vi "1-Continuous B sweep.vi"(2 "Comments":string="SA03036H\nsweep Vsg:-150m to 700m, 500u steps\nB 7T to -7T\nVbg =-3.9V\nT: 50mK\n\nlockin\n\nI+/-: 4/28 200uV ac+ 250u dc bias, 13Hz\nV1+/-: 3/27\nV2+/- 2/6\nV3+/V3-: 7/8\nVsg: 1\nVbg :26\n\ntc 300ms order 2", 3 "ITX folder":string="4L4Lockinfieldsweep", 5 "Sweep rate (T/min)":dbl=0.028 min=0.0 max=0.2, 6 "error in (no error)":errorcluster, 7 "Simulate/Run":enum16{"simulate mode", "run mode"}(ring)=enum."run mode", 8 "Min (start)":dbl=7.0 min=-8.0 max=8.0, 9 "Max (end)":dbl=-7.0 min=-8.0 max=8.0) -> (0 "error out":errorcluster)   [LabVIEW 2016, in "Transport.lvclass"]
uses:
  Transport.lvclass
  SMOs/SweepControl/SweepControl.lvclass
  C:/Program Files (x86)/National Instruments/LabVIEW 2016/vi.lib/JKI/JKI SMO/SMO/SMO.lvclass
panel:
  in  "IPS VISA resource name":refnum<visa-resource-name>="GPIB1::24::INSTR"
  in  "function":enum16{"Ramp", "Triangle", "Sine"}(ring)
  in  "phase":dbl
  in  "cycles (1,2,...)":i32=1 min=1 step=1
  in  "step size":dbl=14.0 format="%.4f"
  out "listener":bool
  out "notifier":bool
  out "B Field Values":dbl[](graph)=[7.0, -7.0]
  in  "Measurement type":enum16{"lockin_Vsg", "lockin_time", "IV"}(ring)
  in  "stop":bool
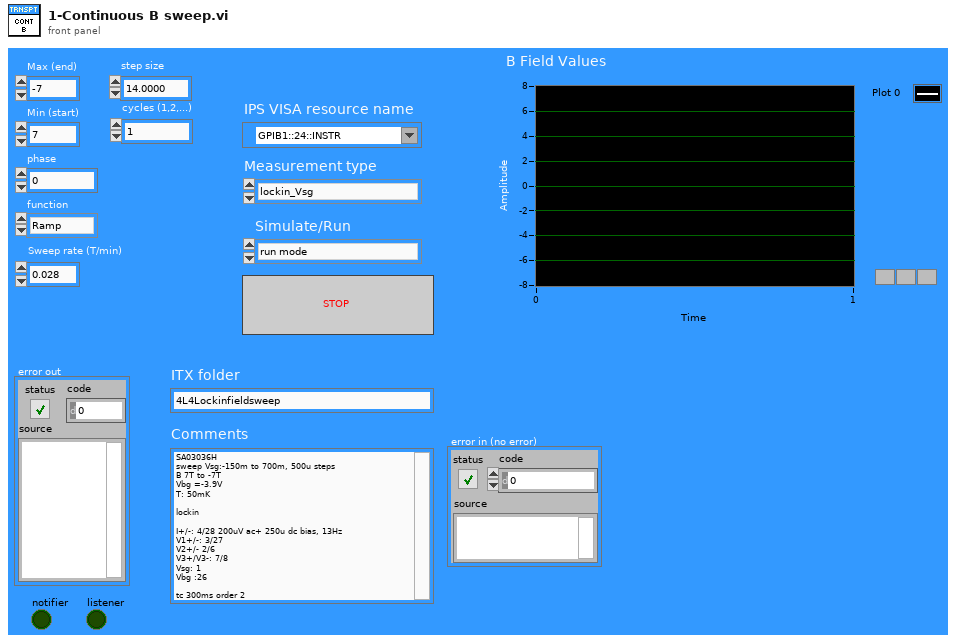
[diagram p1: front panel]
types:
  T1 = cluster{"Target Field (T)":dbl, "Target Field Rate (T/min)":dbl}
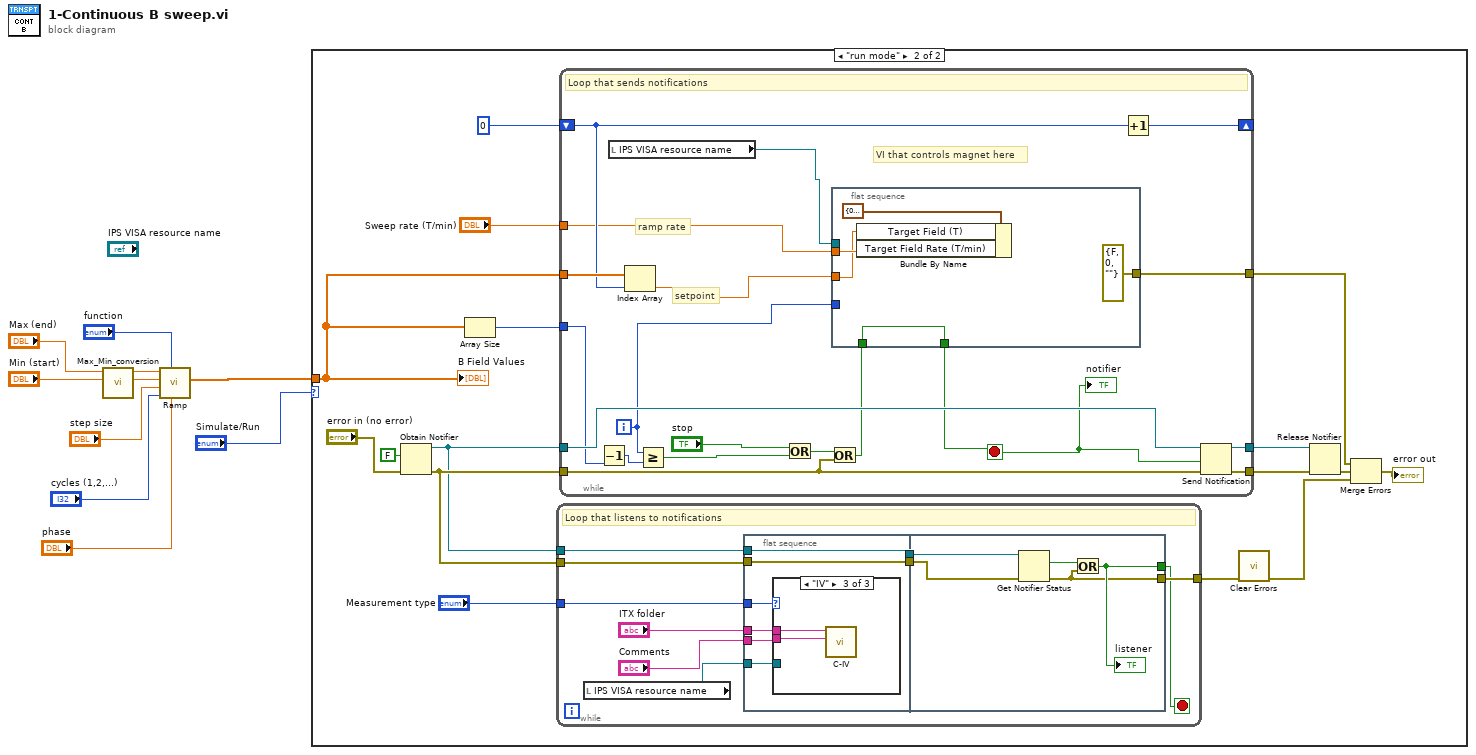
[diagram p0: block diagram]
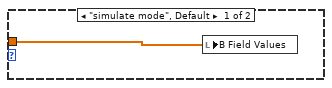
[diagram p2: hidden frame]
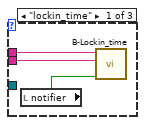
[diagram p3: hidden frame]
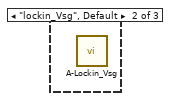
[diagram p4: hidden frame]
diagram:
  n1 = call <userlib>:"Max_Min_conversion.vi"("Min"="Min (start)", "Max"="Max (end)") -> ("offset"=w9:dbl, "Amplitude"=w10:dbl)  [unwired: 8 in]
  n2 = call <userlib>:"Ramp.vi"("phase"="phase", "function (ramp)"="function", "cycles (1,2,...)"="cycles (1,2,...)", "step size"="step size", "offset"=w9, "amplitude"=w10) -> ("Waveform Graph"=w1:dbl[])  [unwired: 3 in, 2 out]
  n3 = case shown="\"run mode\"" "Simulate/Run" {
    tunnel: w1 -> [w11 w14]
    frame "simulate mode", Default {
      n4 = local write "B Field Values"(w11) -> ()
    }
    frame "run mode" {
      n5 = Obtain Notifier(notification data type=FALSE, error in (no error)="error in (no error)") -> (notifier out=w26:refnum<notifier>, error out=w27:errorcluster)  [unwired: 2 in, 1 out]
      n6 = Array Size(array=w14) -> (size(s)=w15:i32)
      n7 = while {
        tunnel: w27 -> [w33]
        tunnel: w26 -> [w35]
        tunnel: "Measurement type" -> [w37]
        tunnel: [w32] -> w16
        stop <- w31 stop-if-true
        # "Loop that listens to notifications"
        n8 = local read "IPS VISA resource name"() -> (w28:refnum<visa-resource-name>)
        n9 = flat-sequence {
          tunnel: w37 -> [w39]
          tunnel: "ITX folder" -> [w43]
          tunnel: "Comments" -> [w42]
          tunnel: [w41] -> w36
          tunnel: w35 -> [w41]
          tunnel: [w40] -> w34
          tunnel: w33 -> [w40]
          tunnel: w28 -> [w38]
          tunnel: w36 -> [w53]
          tunnel: w34 -> [w52]
          tunnel: [w51] -> w31
          tunnel: [w50] -> w32
          frame #0 {
            n10 = case shown="\"IV\"" w39 {
              tunnel: w43 -> [w46 _ w48]
              tunnel: w42 -> [w45 _ w47]
              tunnel: w38 -> [_ _ _]
              frame "lockin_time" {
                n11 = local read "notifier"() -> (w44:bool)
                n12 = call "B-Lockin_time.vi"("stop"=w44, "Comments"=w45, "folder name"=w46) -> ()  [unwired: 6 in, 3 out]
              }
              frame "lockin_Vsg", Default {
                n13 = call "A-Lockin_Vsg.vi"() -> ()  [unwired: 11 in, 1 out]
              }
              frame "IV" {
                n14 = call "C-IV.vi"(10:w47, "SweepControl.lvclass"=w48) -> ()  [unwired: 9 in, 1 out]
              }
            }
          }
          frame #1 {
            n15 = Get Notifier Status(notifier=w53, error in (no error)=w52) -> (current notification=w49:bool, error out=w50:errorcluster)  [unwired: 3 out]
            n16 = Or(x=w49, y=w50) -> (x .or. y?=w51:bool)
            "listener" <- w51
          }
        }
      }
      n17 = while {
        tunnel: w26 -> [w70]
        tunnel: w27 -> [w67]
        tunnel: [w72] -> w17
        tunnel: [w71] -> w25
        tunnel: "Sweep rate (T/min)" -> [w54]
        shift-right: [w66] -> _
        shift-left: 0 -> [w61]
        tunnel: w14 -> [w65]
        tunnel: w15 -> [w62]
        tunnel: [w55] -> w12
        i -> [w59]
        stop <- w56 stop-if-true
        # "VI that controls magnet here"
        # "setpoint"
        # "ramp rate"
        # "Loop that sends notifications"
        n18 = Decrement(x=w62) -> (x-1=w63:i32)
        n19 = local read "IPS VISA resource name"() -> (w58:refnum<visa-resource-name>)
        n20 = Index Array(array=w65, index=w61) -> (element=w60:dbl)
        n21 = Greater Or Equal?(x=w59, y=w63) -> (x >= y?=w64:bool)
        n22 = Or(x="stop", y=w64) -> (x .or. y?=w68:bool)
        n23 = Or(x=w68, y=w67) -> (x .or. y?=w57:bool)
        n24 = flat-sequence {
          tunnel: w54 -> [w75]
          tunnel: w60 -> [w74]
          tunnel: w59 -> [_]
          tunnel: w58 -> [_]
          tunnel: w57 -> [w77]
          tunnel: [w77] -> w56
          tunnel: [errorcluster {"status"=FALSE, "code"=0, "source"=""} ("error out")] -> w55
          frame #0 {
            n25 = Bundle By Name(cluster=T1 {"Target Field (T)"=0.1, "Target Field Rate (T/min)"=0.1} ("IPS120 Targets"), "Target Field (T)"=w74, "Target Field Rate (T/min)"=w75) -> ()  [unwired: 1 out]
          }
        }
        n26 = Increment(x=w61) -> (x+1=w66:i32)
        n27 = Send Notification(notification=w56, notifier=w70, error in (no error)=w67) -> (notifier out=w72:refnum<notifier>, error out=w71:errorcluster)
        "notifier" <- w56
      }
      n28 = call <vilib>:"Clear Errors.vi"("error in (no error)"=w16) -> ("error out"=w13:errorcluster)  [unwired: 5 in, 1 out]
      n29 = Release Notifier(notifier=w17, error in (no error)=w25) -> (error out=w19:errorcluster)  [unwired: 1 in, 2 out]
      n30 = Merge Errors(w12, w19, w13) -> (→"error out":errorcluster)
      "B Field Values" <- w14
    }
  }
